vi "Set Menu Coordinates.vi"(6 "Position":T1, 8 "error in (no error)":errorcluster, 10 "HamburgerCtl Ref":refnum<vi>, 11 "VI in":refnum<vi>) -> (0 "error out":errorcluster, 3 "VI out":refnum<vi>)   [LabVIEW 2017, in "Hamburger Menu Library.lvlib"]
uses:
  Hamburger Menu Library.lvlib
  Menu Position.ctl
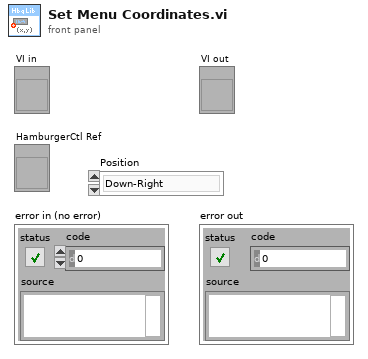
[diagram p1: front panel]
types:
  T1 = typedef "Hamburger Menu Library.lvlib/Menu Position.ctl" = enum16{"Down-Right", "Down-Left"}
  T2 = enum32{"Invalid", "Standard", "Closed", "Hidden", "Minimized", "Maximized"}
  T3 = typedef "LVRectTypeDef.ctl" = cluster{"Left":i16, "Top":i16, "Right":i16, "Bottom":i16}
  T4 = typedef "LVBoundsTypeDef.ctl" = cluster{"Width":u32, "Height":u32}
  T5 = typedef "LVPositionTypeDef.ctl" = cluster{"Left":i32, "Top":i32}
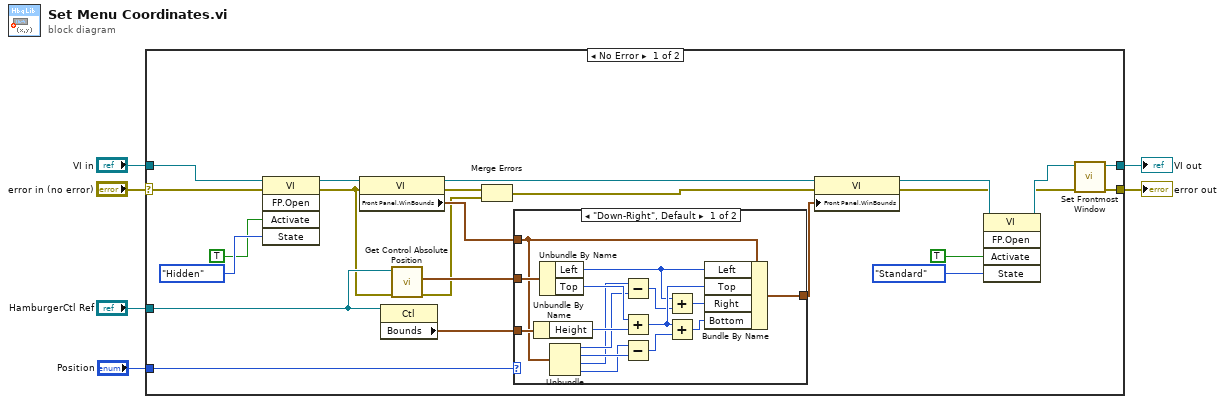
[diagram p0: block diagram]
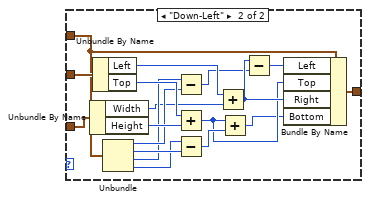
[diagram p2: hidden frame]
diagram:
  n1 = case shown="No Error" "error in (no error)" {
    selector: "error in (no error)" -> [w10 w66]
    tunnel: [w30 w65] -> w5
    tunnel: [w29 w66] -> w4
    tunnel: "HamburgerCtl Ref" -> [w23 _]
    tunnel: "VI in" -> [w11 w65]
    tunnel: "Position" -> [w7 _]
    frame No Error {
      n2 = invoke class="VI" method="FP.Open"(reference=w11, error in=w10, "Activate"=TRUE ("Activate?"), "State"=T2."Hidden") -> (reference out=w8:refnum<vi>, error out=w9:errorcluster)  [unwired: 1 in, 3 out]
      n3 = property class="VI"(reference=w8, error in=w9) -> (reference out=w28:refnum<vi>, error out=w22:errorcluster, "Front Panel.WinBounds"=w24:T3)
      n4 = property class="Ctl"(reference=w23) -> ("Bounds"=w26:T4)  [unwired: 1 in, 2 out]
      n5 = call "Get Control Absolute Position.vi"("error in (no error)"=w9, "Boolean in"=w23) -> ("error out"=w21:errorcluster, "Absolute Position"=w25:T5)  [unwired: 8 in]
      n6 = Merge Errors(w22, w21) -> (w20:errorcluster)
      n7 = case shown="\"Down-Right\", Default" w7 {
        tunnel: [w46 w64] -> w27
        tunnel: w26 -> [w37 w60]
        tunnel: w25 -> [w36 w59]
        tunnel: w24 -> [w31 w54]
        frame "Down-Right", Default {
          n8 = Unbundle By Name(w37) -> ("Height"=w39:u32)
          n9 = Unbundle By Name(w36) -> ("Left"=w40:i32, "Top"=w38:i32)
          n10 = Unbundle(w31) -> ("Left"=w33:i16, "Top"=w35:i16, "Right"=w32:i16, "Bottom"=w34:i16)
          n11 = Subtract(x=w32, y=w33) -> (x-y=w41:i16)
          n12 = Add(x=w38, y=w39) -> (x+y=w43:u32)
          n13 = Subtract(x=w34, y=w35) -> (x-y=w44:i16)
          n14 = Add(x=w40, y=w41) -> (x+y=w42:i32)
          n15 = Add(x=w43, y=w44) -> (x+y=w45:u32)
          n16 = Bundle By Name(cluster=w31, "Left"=w40, "Top"=w43, "Right"=w42, "Bottom"=w45) -> (w46:T3)
        }
        frame "Down-Left" {
          n17 = Unbundle By Name(w60) -> ("Width"=w52:u32, "Height"=w62:u32)
          n18 = Unbundle By Name(w59) -> ("Left"=w53:i32, "Top"=w61:i32)
          n19 = Unbundle(w54) -> ("Left"=w56:i16, "Top"=w58:i16, "Right"=w55:i16, "Bottom"=w57:i16)
          n20 = Subtract(x=w55, y=w56) -> (x-y=w50:i16)
          n21 = Add(x=w61, y=w62) -> (x+y=w48:u32)
          n22 = Subtract(x=w57, y=w58) -> (x-y=w63:i16)
          n23 = Add(x=w53, y=w52) -> (x+y=w51:u32)
          n24 = Add(x=w48, y=w63) -> (x+y=w47:u32)
          n25 = Subtract(x=w51, y=w50) -> (x-y=w49:u32)
          n26 = Bundle By Name(cluster=w54, "Left"=w49, "Top"=w48, "Right"=w51, "Bottom"=w47) -> (w64:T3)
        }
      }
      n27 = property class="VI"(reference=w28, error in=w20, "Front Panel.WinBounds"=w27) -> (reference out=w19:refnum<vi>, error out=w14:errorcluster)
      n28 = invoke class="VI" method="FP.Open"(reference=w19, error in=w14, "Activate"=TRUE ("Activate?"), "State"=T2."Standard") -> (reference out=w16:refnum<vi>, error out=w15:errorcluster)  [unwired: 1 in, 3 out]
      n29 = call "Set Frontmost Window.vi"("error in (no error)"=w15, "VI in"=w16) -> ("error out"=w29:errorcluster, "VI out"=w30:refnum<vi>)  [unwired: 8 in]
    }
    frame Error {
    }
  }
  "VI out" <- w5
  "error out" <- w4
